vi "Last Aperture Time Getter.vi"(11 "error in (no error)":errorcluster) -> (4 "Aperture Time (s)":dbl, 15 "error out":errorcluster)   [LabVIEW 2023, in "NI-568x RF Power Meter.lvlib" / "SG 2250 Path Accessor.lvclass"]
uses:
  SG 2250 Path Accessor.lvclass
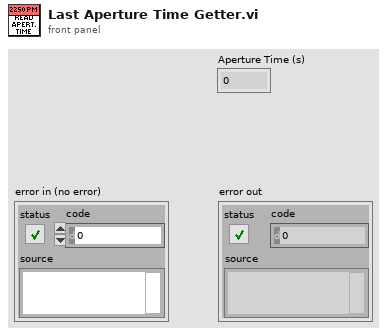
[diagram p1: front panel]
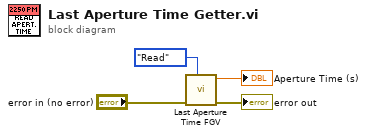
[diagram p0: block diagram]
diagram:
  n1 = call "Last Aperture Time FGV.vi"("Action"=enum16{"Write", "Read"}."Read", "error in (no error)"="error in (no error)") -> ("error out"=→"error out":errorcluster, "Aperture Time (s)"=→"Aperture Time (s)":dbl)  [unwired: 5 in]
